vi "Variable list Tool analog.vi"() -> (6 "Variant":variant, 10 "Array":T1[](array[typedef]) {"Default Scaling"."Offset" format="%.5f"; "Default Scaling"."Gain" format="%.5f"})   [LabVIEW 2011]
uses:
  Measurments Handling/Fixed Analog Channel Definition.ctl
  Measurments Handling/Units/Quantity enum.ctl
  Measurments Handling/Update frequensies.ctl
  Measurments Handling/Channel catagory Enum.ctl
  Measurments Handling/Scaling.ctl
  Measurments Handling/Channel Classification Enum.ctl
  Variable List Tool Analog.ctl
  Measurments Handling/Common/Variable List Common Analog.ctl
  <vilib>/Utility/VariantDataType/GetNumericInfo.vi
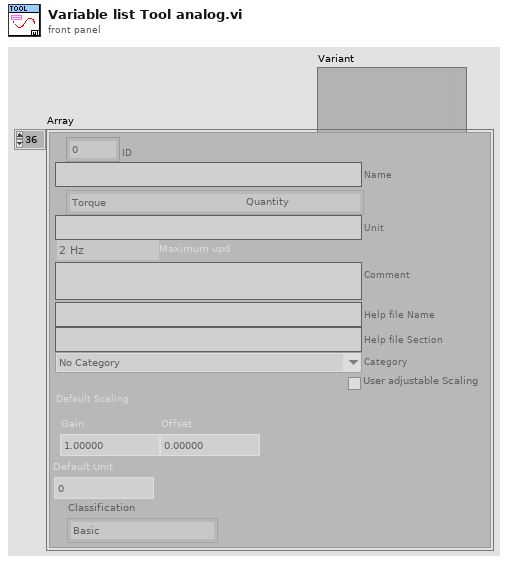
[diagram p1: front panel]
types:
  T1 = typedef "Fixed Analog Channel Definition.ctl" = cluster{"ID":u16, "Name":string, "Quantity":T2, "Unit":string, "Maximum upd":T3, "Comment":string, "Help file Name":string, "Help file Section ":string, "Category":T4, "User adjustable Scaling":bool, "Default Scaling":T5, "Default Unit":i32, "Classification":T6}
  T2 = typedef "Quantity enum.ctl" = enum16{"NA", "Acceleration", "Angle", "Current", "Force", "Distance", "Pressure", "Resistance", "Rotational Speed", "Speed", "Temperature", "Tension", "Torque", "Voltage", "Weight"}
  T3 = typedef "Update frequensies.ctl" = enum16{"2 Hz", "1 Hz", "0.1 Hz"}
  T4 = typedef "Channel catagory Enum.ctl" = enum16{"No Category", "Power", "Temperature", "Pressure"}
  T5 = typedef "Scaling.ctl" = cluster{"Gain":dbl, "Offset":dbl}
  T6 = typedef "Channel Classification Enum.ctl" = enum16{"Basic", "Advanced", "Expert", "Unused"}
  T7 = typedef "Variable List Common Analog.ctl" = enum16{"HVPSU Head Voltage", "HVPSU TS Voltage", "HVPSU Current", "PCP Cable Resistance", "Winch Depth", "Winch Line Speed", "Winch Wire Tension"}
  T8 = typedef "Variable List Tool Analog.ctl" = enum16{"Tool Max Temperature", "Tool (Controller) Temperature", "Tool Supply Voltage", "Tool (Controller) Current", "Tool Acceleration X", "Tool Acceleration Y", "Tool Acceleration Z", "Tool Acceleration Sum", "Tool Inclination", "Tool Rotation", "Tool GP Sensor 1", "Tool GP Sensor 2", "Tool (Pressure 1) Temperature", "Tool Pressure 1 RAW", "Tool (Pressure 2) Temperature", "Tool Pressure 2 RAW", "Tool (Solenoid) Temperature", "Tool Solenoid Position", "PSU Temp", "Head Voltage", "PSU Main Voltage out", "PSU Main Current out", "Upper Tension Sub Temp", "Tool Upper Tension Sub Raw", "Lower Tension Sub Temp", "Tool Lower Tension Sub Raw", "Tool Var27 - Reserved", "Tool Var28 - Reserved", "Tool Var29 - Reserved", "Tool Var30 - Reserved", "Stroke Extension", "Stroke In Force", "Stroke Out Force", "Stroke Force", "Stroker Pressure 1", "Stroker Pressure 2", "Stroker Upper Tension Sub", "Stroker Lower Tension Sub", "Stroker Var09 - Reserved", "Stroker Var10 - Reserved", "Tractor Upper Tension Sub", "Tractor Lower Tension Sub", "Tractor Var03 - Reserved", "Tractor Var04 - Reserved", "Tool Temperature sensor", "Tool Motor Voltage", "Tool Motor Current", "Tool Motor Torque", "Tool weight on bit", "Tool Motor RPM"}
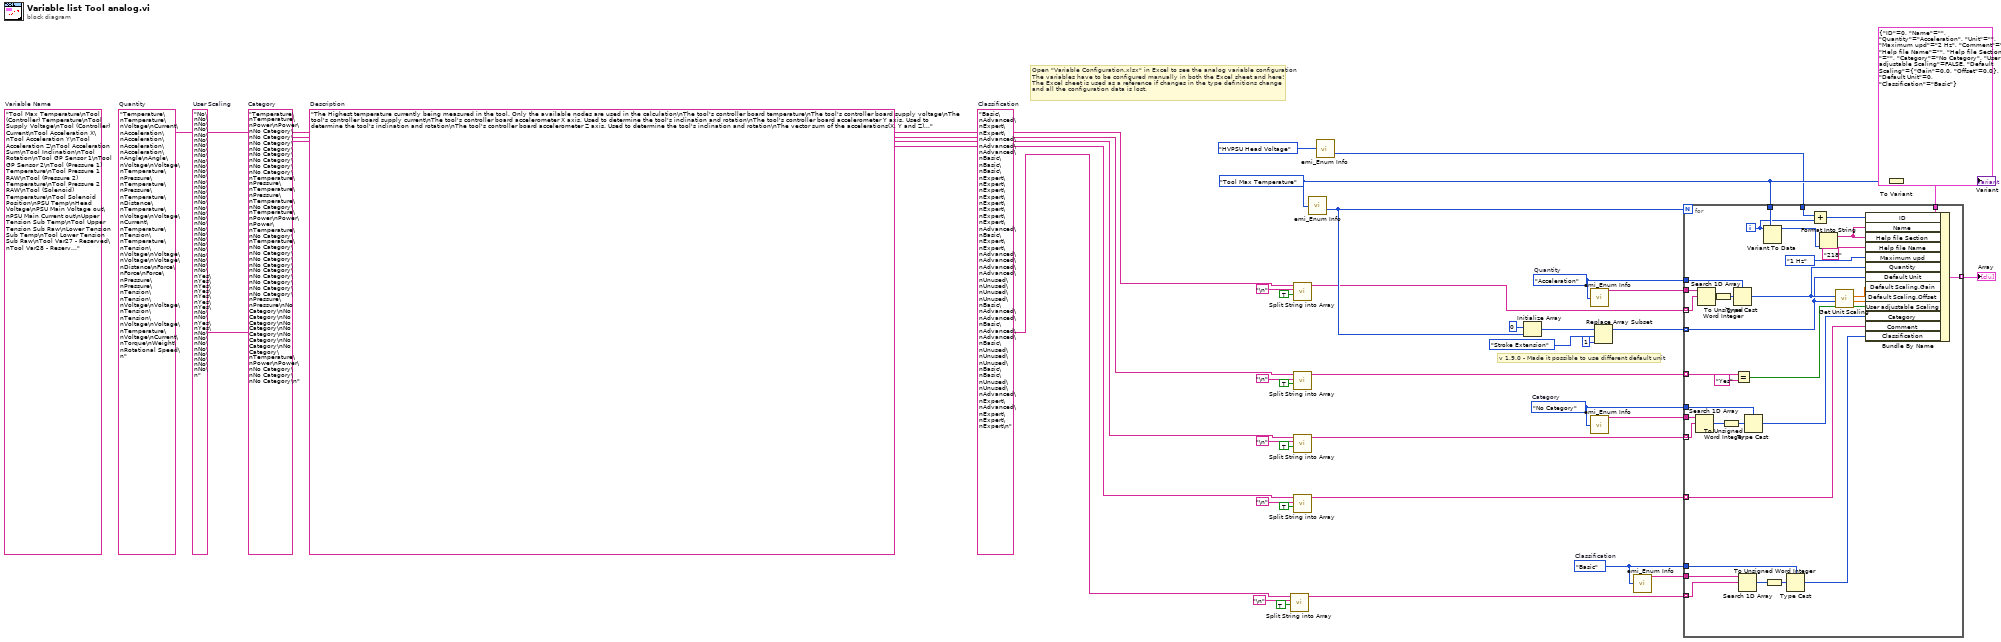
[diagram p0: block diagram]
diagram:
  w3 = Channel_Classification_Enum."Basic"  # Classification
  w4 = "Basic\nAdvanced\nExpert\nExpert\nAdvanced\nAdvanced\nAdvanced\nBasic\nBasic\nBasic\nExpert\nExpert\nExpert\nExpert\nExpert\nExpert\nExpert\nExpert\nAdvanced\nBasic\nExpert\nExpert\nAdvanced\nAdvanced\nAdvanced\nAdvanced\nUnused\nUnused\nUnused\nUnused\nBasic\nAdvanced\nAdvanced\nBasic\nAdvanced\nAdvanced\nBasic\nUnused\nUnused\nUnused\nBasic\nBasic\nUnused\nUnused\nAdvanced\nExpert\nAdvanced\nExpert\nExpert\nExpert\n"  # Classification
  w11 = "Temperature\nTemperature\nPower\nPower\nNo Category\nNo Category\nNo Category\nNo Category\nNo Category\nNo Category\nNo Category\nNo Category\nTemperature\nPressure\nTemperature\nPressure\nTemperature\nNo Category\nTemperature\nPower\nPower\nPower\nTemperature\nNo Category\nTemperature\nNo Category\nNo Category\nNo Category\nNo Category\nNo Category\nNo Category\nNo Category\nNo Category\nNo Category\nPressure\nPressure\nNo Category\nNo Category\nNo Category\nNo Category\nNo Category\nNo Category\nNo Category\nNo Category\nTemperature\nPower\nPower\nNo Category\nNo Category\nNo Category\n"  # Category
  w14 = Channel_catagory_Enum."No Category"  # Category
  w17 = "No\nNo\nNo\nNo\nNo\nNo\nNo\nNo\nNo\nNo\nNo\nNo\nNo\nNo\nNo\nNo\nNo\nNo\nNo\nNo\nNo\nNo\nNo\nNo\nNo\nNo\nNo\nNo\nNo\nNo\nNo\nYes\nYes\nYes\nYes\nYes\nYes\nYes\nNo\nNo\nYes\nYes\nNo\nNo\nNo\nNo\nNo\nNo\nNo\nNo\n"  # User Scaling
  w22 = Quantity_enum."Acceleration"  # Quantity
  w9 = "Temperature\nTemperature\nVoltage\nCurrent\nAcceleration\nAcceleration\nAcceleration\nAcceleration\nAngle\nAngle\nVoltage\nVoltage\nTemperature\nPressure\nTemperature\nPressure\nTemperature\nDistance\nTemperature\nVoltage\nVoltage\nCurrent\nTemperature\nTension\nTemperature\nTension\nVoltage\nVoltage\nVoltage\nVoltage\nDistance\nForce\nForce\nForce\nPressure\nPressure\nTension\nTension\nVoltage\nVoltage\nTension\nTension\nVoltage\nVoltage\nTemperature\nVoltage\nCurrent\nTorque\nWeight\nRotational Speed\n"  # Quantity
  w21 = "The Highest temperature currently being measured in the tool. Only the available nodes are used in the calculation\nThe tool's controller board temperature\nThe tool's controller board supply voltage\nThe tool's controller board supply current\nThe tool's controller board accelerometer X axis. Used to determine the tool's inclination and rotation\nThe tool's controller board accelerometer Y axis. Used to determine the tool's inclination and rotation\nThe tool's controller board accelerometer Z axis. Used to determine the tool's inclination and rotation\nThe vector sum of the accelerations(X, Y and Z) measured on the tool's controller board\nThe tools inclination, as calculated by the accelerations (X, Y and Z) measured on the tool's controller board. 0deg indicates straight down, 180deg indicates straight up, 90deg is level\nThe tools rotation, as calculated by the accelerations (X, Y and Z) measured on the tool's controller board. This is not calculated if the inclination is within 10 deg of 0 deg or 180 deg\nTool's controller board 24bit analog input bridge sensor no 1\nTool's controller board 24bit analog input bridge sensor no 2\nTemperature measured at pressure node 1 in the tool\nUnscaled pressure measured by pressure node 1  in the tool\nTemperature measured by pressure node 2  in the tool\nUnscaled pressure measured by pressure node 2 in the tool\nTemperature of the Solenoid electronics\nUnscaled value of Solenoid position\nTemperature measured in PSU\nInput voltage of PSU\nOutput voltage of PSU\nOutput current of PSU\nTemperature measured at the upper tension sub node in the tool\nUnscaled tension measured by the upper tension sub node in the tool\nTemperature measured at the lower tension sub node in the tool\nUnscaled tension measured by the lower tension sub node in the tool\nReserved for future expansion\nReserved for future expansion\nReserved for future expansion\nReserved for future expansion\nHow far the tool's stroke is extending from its retracted position\nThe stroke in force as measured by the pressure transmitter. (Pressure * 0.0197)\nThe stroke out force as measured by the pressure transmitter. (Pressure * 0.0197)\nTotal stroke force. The difference between the pressures measured at the two pressure nodes, is multiplied by 0.0197 tonnes. The pressure of Node 2 is subtracted from the pressure of Node 1.\nStroker pressure measured by pressure node 1 in the tool\nStroker pressure measured by pressure node 1 in the tool\nStroker tension measured by the upper tension sub node in the tool\nStroker tension measured by the lower tension sub node in the tool\nReserved for future expansion\nReserved for future expansion\nTractor tension measured by the upper tension sub node in the tool\nTractor tension measured by the lower tension sub node in the tool\nReserved for future expansion\nReserved for future expansion\nTool dedicated temperature sensor\nMotor voltage\nCurrent measured at motor driver\nTorque calculated from motor current and voltage\nTool weight on bit\nRotational speed of bit\n"  # Description
  (unwired) "Tool Max Temperature\nTool (Controller) Temperature\nTool Supply Voltage\nTool (Controller) Current\nTool Acceleration X\nTool Acceleration Y\nTool Acceleration Z\nTool Acceleration Sum\nTool Inclination\nTool Rotation\nTool GP Sensor 1\nTool GP Sensor 2\nTool (Pressure 1) Temperature\nTool Pressure 1 RAW\nTool (Pressure 2) Temperature\nTool Pressure 2 RAW\nTool (Solenoid) Temperature\nTool Solenoid Position\nPSU Temp\nHead Voltage\nPSU Main Voltage out\nPSU Main Current out\nUpper Tension Sub Temp\nTool Upper Tension Sub Raw\nLower Tension Sub Temp\nTool Lower Tension Sub Raw\nTool Var27 - Reserved\nTool Var28 - Reserved\nTool Var29 - Reserved\nTool Var30 - Reserved\nStroke Extension\nStroke In Force\nStroke Out Force\nStroke Force\nStroker Pressure 1\nStroker Pressure 2\nStroker Upper Tension Sub\nStroker Lower Tension Sub\nStroker Var09 - Reserved\nStroker Var10 - Reserved\nTractor Upper Tension Sub\nTractor Lower Tension Sub\nTractor Var03 - Reserved\nTractor Var04 - Reserved\nTool Temperature sensor\nTool Motor Voltage\nTool Motor Current\nTool Motor Torque\nTool weight on bit\nTool Motor RPM\n"  # Variable Name
  w35 = Variable_List_Tool_Analog."Tool Max Temperature" ("Variable ID")
  # "v 1.9.0 - Made it possible to use different default unit"
  # "Open \"Variable Configuration.xlsx\" in Excel to see the analog variable configuration\nThe variables have to be configured manually in both the Excel sheet and here!\nThe Excel sheet is used as a reference if changes in the type definitions change\nand all the configuration data is lost."
  n1 = call "Split String into Array.vi"("Remove Last Row"=TRUE, "Separator"="\n", "Input string"=w4) -> ("Array of cells"=w1:string[])  [unwired: 8 in]
  n2 = call "Split String into Array.vi"("Remove Last Row"=TRUE, "Separator"="\n", "Input string"=w9) -> ("Array of cells"=w24:string[])  [unwired: 8 in]
  n3 = call "Split String into Array.vi"("Remove Last Row"=TRUE, "Separator"="\n", "Input string"=w17) -> ("Array of cells"=w16:string[])  [unwired: 8 in]
  n4 = call "Split String into Array.vi"("Remove Last Row"=TRUE, "Separator"="\n", "Input string"=w11) -> ("Array of cells"=w10:string[])  [unwired: 8 in]
  n5 = call "Split String into Array.vi"("Remove Last Row"=TRUE, "Separator"="\n", "Input string"=w21) -> ("Array of cells"=w20:string[])  [unwired: 8 in]
  n6 = call "emi_Enum Info.vi"("Enum"=w35) -> ("Numb Elements"=w34:i32)  [unwired: 11 in, 3 out]
  n7 = call "emi_Enum Info.vi"("Enum"=Variable_List_Common_Analog."HVPSU Head Voltage" ("Action")) -> ("Numb Elements"=w7:i32)  [unwired: 11 in, 3 out]
  n8 = Initialize Array(0, w34) -> (w32:i32[])
  n9 = call "emi_Enum Info.vi"("Enum"=w22) -> ("Text Elements"=w23:string[])  [unwired: 11 in, 3 out]
  n10 = call "emi_Enum Info.vi"("Enum"=w14) -> ("Text Elements"=w15:string[])  [unwired: 11 in, 3 out]
  n11 = Replace Array Subset(array=w32, new element=1 ("new element/subarray"), index=Variable_List_Tool_Analog."Stroke Extension" ("Variable ID")) -> (w30:i32[])
  n12 = call "emi_Enum Info.vi"("Enum"=w3) -> ("Text Elements"=w2:string[])  [unwired: 11 in, 3 out]
  n13 = for {
    N: w34 -> [_]
    tunnel: [w73] -> w36 mode=indexing
    tunnel: T1 {"ID"=0, "Name"="", "Quantity"=enum."Acceleration", "Unit"="", "Maximum upd"=enum."2 Hz", "Comment"="", "Help file Name"="", "Help file Section "="", "Category"=enum."No Category", "User adjustable Scaling"=FALSE, "Default Scaling"={"Gain"=0.0, "Offset"=0.0}, "Default Unit"=0, "Classification"=enum."Basic"} ("Variable Defenition") -> [w72]
    tunnel: w35 -> [w71]
    tunnel: w20 -> [w52] mode=indexing
    tunnel: w30 -> [w59] mode=indexing
    tunnel: w24 -> [w66] mode=indexing
    tunnel: w23 -> [w67]
    tunnel: w22 -> [w64]
    tunnel: w16 -> [w58] mode=indexing
    tunnel: w10 -> [w54] mode=indexing
    tunnel: w15 -> [w53]
    tunnel: w14 -> [w55]
    tunnel: w7 -> [w47]
    tunnel: w1 -> [w41] mode=indexing
    tunnel: w2 -> [w42]
    tunnel: w3 -> [w40]
    i -> [w46]
    n14 = Search 1D Array(1D array=w53, element=w54) -> (index of element=w50:i32)  [unwired: 1 in]
    n15 = Search 1D Array(1D array=w67, element=w66) -> (index of element=w65:i32)  [unwired: 1 in]
    n16 = To Unsigned Word Integer(number=w65) -> (unsigned 16bit integer=w48:u16)
    n17 = To Unsigned Word Integer(number=w50) -> (unsigned 16bit integer=w49:u16)
    n18 = Type Cast(type=w64, x=w48) -> (*(type *) &x=w62:T2)
    n19 = Equal?(x=w58, y="Yes") -> (x = y?=w56:bool)
    n20 = Search 1D Array(1D array=w42, element=w41) -> (index of element=w43:i32)  [unwired: 1 in]
    n21 = Type Cast(type=w55, x=w49) -> (*(type *) &x=w51:T4)
    n22 = Variant To Data(type=w71, Variant=w46) -> (data=w70:T8)  [unwired: 1 in, 1 out]
    n23 = To Unsigned Word Integer(number=w43) -> (unsigned 16bit integer=w44:u16)
    n24 = Type Cast(type=w40, x=w44) -> (*(type *) &x=w39:T6)
    n25 = Add(x=w47, y=w46) -> (x+y=w45:i32)
    n26 = Format Into String(w70) -> (resulting string=w69:string)  [unwired: 3 in, 1 out]
    n27 = call "Get Unit Scaling.vi"("Unit Index"=w59, "Quantity"=w62) -> ("Offset"=w60:dbl, "Gain"=w61:dbl)  [unwired: 7 in, 1 out]
    n28 = Bundle By Name(cluster=w72, "ID"=w45, "Name"=w69, "Help file Section"=w69, "Help file Name"="218", "Maximum upd"=Update_frequensies."1 Hz", "Quantity"=w62, "Default Unit"=w59, "Default Scaling.Gain"=w61, "Default Scaling.Offset"=w60, "User adjustable Scaling"=w56, "Category"=w51, "Comment"=w52, "Classification"=w39) -> (w73:T1)
  }
  "Array" <- w36
  n29 = To Variant(anything=w35) -> (Variant=→"Variant":variant)
